vi "All Channels.vi"(8 "error in (no error)":errorcluster, 11 "Group in":refnum<class "Group.lvclass">) -> (0 "error out":errorcluster, 2 "All Channels":refnum<class "Channel.lvclass">[](array[class]), 3 "Group out":refnum<class "Group.lvclass">)   [LabVIEW 2020, in "Vecto.lvlib" / "Group.lvclass"]
uses:
  Group.lvclass
  C:/dev/lv20CE/relink/lv-vecto/Vecto/GroupAbstract/GroupAbstract.lvclass
  Channel/Channel.lvclass
  GroupAbstract/GroupAbstract.lvclass/GroupAbstract.ctl
  Channel/Channel.lvclass/Channel.ctl
  Group Config/Get Channels.vi
  Group.lvclass/Group.ctl
  GroupAbstract/GroupAbstract.lvclass
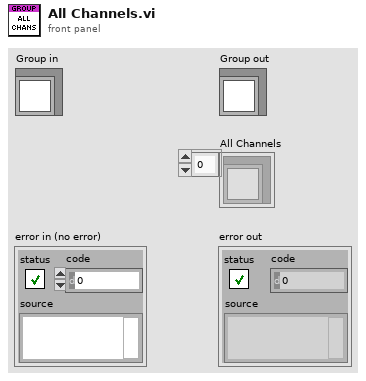
[diagram p1: front panel]
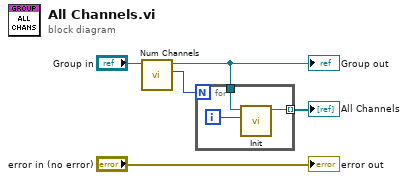
[diagram p0: block diagram]
diagram:
  n1 = call "Num Channels.vi"("GroupAbstract in"="Group in") -> ("Num Channels"=w1:i32, "GroupAbstract out"=w2:refnum<class "Group.lvclass">)  [unwired: 8 in, 1 out]
  "Group out" <- w2
  n2 = for {
    N: w1 -> [_]
    tunnel: w2 -> [w7]
    tunnel: [w6] -> w4 mode=indexing
    i -> [w8]
    n3 = call "Init.vi"("Channel Index"=w8, "Group"=w7) -> ("Channel out"=w6:refnum<class "Channel.lvclass">)  [unwired: 8 in, 1 out]
  }
  "All Channels" <- w4
  "error out" <- "error in (no error)"
